vi "Look in Map.vi"(8 "error in":errorcluster, 10 "key":string, 11 "map":map{string, i32}(c390)) -> (0 "error out":errorcluster, 3 "value":i32)   [LabVIEW 2024]
uses:
  Configure Strategies/DAQmx/DAQmx Thermocouple Continuous Read Strategy/DAQmx Thermocouple Continuous Read Strategy.lvclass/DAQmx Thermocouple Continuous Read Strategy.ctl
  Configure Strategies/DAQmx/DAQmx Thermocouple Continuous Read Strategy/DAQmx Thermocouple Continuous Read Strategy.lvclass
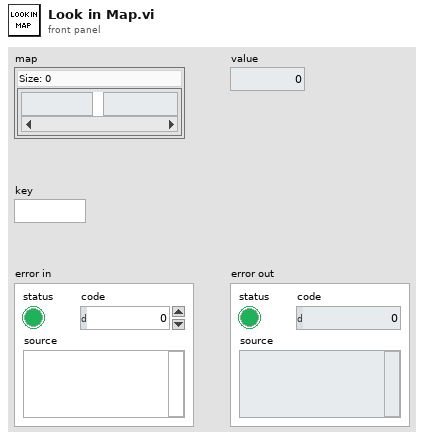
[diagram p1: front panel]
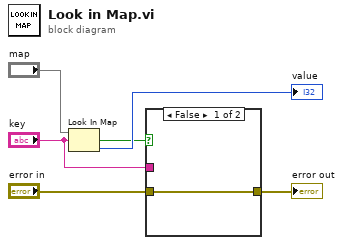
[diagram p0: block diagram]
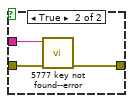
[diagram p2: hidden frame]
diagram:
  n1 = Look In Map(map="map", key="key") -> (key not found?=w4:bool, value=→"value":i32)  [unwired: 1 in]
  n2 = case shown="False" w4 {
    tunnel: [w7 w9] -> w3
    tunnel: "error in" -> [w7 w10]
    tunnel: "key" -> [_ w8]
    frame False {
    }
    frame True {
      n3 = call "5777 key not found--error.vi"("error in"=w10, "Argument"=w8) -> ("error out"=w9:errorcluster)  [unwired: 8 in, 1 out]
    }
  }
  "error out" <- w3
